vi "校准流程.vi"(0 "校准模式":T3(ring), 5 "参数下拉列表":u16(ring) items=["总氮"=1, "总磷"=2], 7 "测量模式":T1(ring), 9 "量程下拉列表":enum16{"低量程", "高量程"}(ring), 11 "曲线模型":T2={"标液浓度1"=0.0, "测量吸光度1"=0.0, "样品1启用"=FALSE, "标液浓度2"=0.0, "测量吸光度2"=0.0, "样品2启用"=FALSE, "标液浓度3"=0.0, "测量吸光度3"=0.0, "样品3启用"=FALSE, "标液浓度4"=0.0, "测量吸光度4"=0.0, "样品4启用"=FALSE, "标液浓度5"=0.0, "测量吸光度5"=0.0, "样品5启用"=FALSE, "模型"=enum."线性", "精度"=4.0, "XY图"=[], "拟合公式"="", "r^2"=0.0, "标样一校准时间"=timestamp(0 s since 1904-01-01), "标样二校准时间"=timestamp(0 s since 1904-01-01), "标样三校准时间"=timestamp(0 s since 1904-01-01), "标样四校准时间"=timestamp(0 s since 1904-01-01), "标样五校准时间"=timestamp(0 s since 1904-01-01), "二次方程"={"c"=0.0, "x"=0.0, "x^2"=0.0}, "标定时间"=timestamp(0 s since 1904-01-01)} {"标定时间" format="%<%m/%d/%y %H:%M:%S>T"; "标样五校准时间" format="%<%m/%d/%y %H:%M:%S>T"; "标样四校准时间" format="%<%m/%d/%y %H:%M:%S>T"; "标样三校准时间" format="%<%m/%d/%y %H:%M:%S>T"; "标样二校准时间" format="%<%m/%d/%y %H:%M:%S>T"; "标样一校准时间" format="%<%m/%d/%y %H:%M:%S>T"; "r^2" format="%.7f"; "测量吸光度5" format="%#.6f"; "测量吸光度4" format="%#.6f"; "测量吸光度3" format="%#.6f"; "测量吸光度2" format="%#.6f"; "测量吸光度1" format="%#.6f"}) -> ()   [LabVIEW 2016, in "斯坦道总磷.lvlib"]
panel:
  out "输出簇":cluster{"数据时间":timestamp, "X值":sgl}
  # "校准时间"
  # "标液浓度"
  # "吸光值显示"
  # "标液一"
  # "标液二"
  # "标液三"
  # "零点"
  # "跨度"
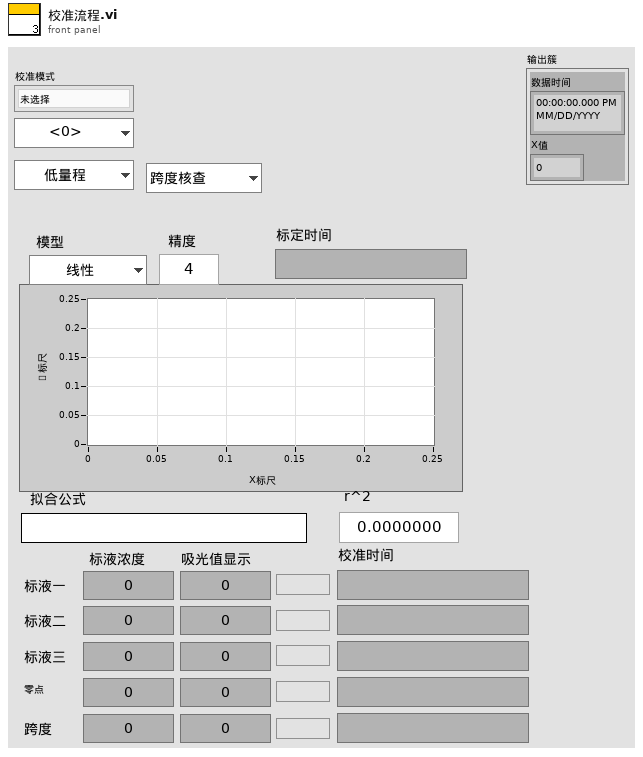
[diagram p1: front panel]
types:
  T1 = enum16{"跨度核查", "水样测量", "零点核查", "标样核查", "加标回收", "快捷测试", "空白校准", "标样校准"}
  T2 = cluster{"标液浓度1":dbl, "测量吸光度1":dbl, "样品1启用":bool, "标液浓度2":dbl, "测量吸光度2":dbl, "样品2启用":bool, "标液浓度3":dbl, "测量吸光度3":dbl, "样品3启用":bool, "标液浓度4":dbl, "测量吸光度4":dbl, "样品4启用":bool, "标液浓度5":dbl, "测量吸光度5":dbl, "样品5启用":bool, "模型":enum32{"线性", "多项式"}, "精度":dbl, "XY图":cluster{"X Values":dbl[], "Y Values":dbl[]}[], "拟合公式":string, "r^2":dbl, "标样一校准时间":timestamp, "标样二校准时间":timestamp, "标样三校准时间":timestamp, "标样四校准时间":timestamp, "标样五校准时间":timestamp, "二次方程":cluster{"c":dbl, "x":dbl, "x^2":dbl}, "标定时间":timestamp}
  T3 = enum32{"未选择", "空白校准", "标样校准", "标样核查", "零点核查", "跨度核查"}
  T4 = enum16{"初始化", "校准启动", "校准运行中", "测试结束", "获取校准数据", "填充校准数据", "流程结束"}
  T5 = enum16{"空闲", "初始化", "校准启动", "校准运行中", "测试结束", "获取校准数据", "填充校准数据", "流程结束"}
  T6 = cluster{"站号":u16, "量程切换":enum32{"H", "L", "AUTO"}, "控制命令":enum16{"启动测量", "标样核查", "零点核查", "跨度核查", "空白测试", "平行样测试", "加标回收", "空白校准", "标样校准", "初始化（清洗）", "停止测试", "仪器重启", "校时", "模式设置", "测量间隔设置"}, "模式设置":enum16{"待机", "连续模式", "周期模式", "定点模式", "受控模式", "手动模式"}, "测量间隔":u16}
  T7 = enum16{"启动测量", "标样核查", "零点核查", "跨度核查", "空白测试", "平行样测试", "加标回收", "空白校准", "标样校准", "初始化（清洗）", "停止测试", "仪器重启", "校时", "模式设置", "测量间隔设置"}
  T8 = cluster{"因子编码":u32, "单位":u16, "标样参考值":sgl, "水样数据时间":timestamp, "水样实测值":sgl, "水样数据标识":string, "标样数据时间":timestamp, "标样实测值":sgl, "标样数据标识":string, "空白数据时间":timestamp, "空白实测值":sgl, "空白数据标识":string, "零点核查数据时间":timestamp, "零点核查实测值":sgl, "零点核查数据标识":string, "跨度核查数据时间":timestamp, "跨度核查实测值":sgl, "跨度核查数据标识":string, "加标回收数据时间":timestamp, "加标回收实测值":sgl, "加标回收数据标识":string, "平行样数据时间":timestamp, "平行样实测值":sgl, "平行样数据标识":string, "F0":sgl, "F1":sgl, "F2":sgl, "F3":sgl, "F4":sgl, "F5":sgl, "F6":sgl, "F7":sgl, "温度":sgl, "湿度":sgl, "X值":sgl, "fidrange":u16, "X1值":sgl}
  T9 = cluster{"系统时间":timestamp, "工作状态":u16, "测量模式":enum16{"待机", "连续模式", "周期模式", "定点模式", "受控模式", "手动模式"}, "告警代码":u16, "故障代码":u16, "日志代码":u16, "软件版本":u16, "F0":sgl, "F1":sgl, "F2":sgl, "F3":sgl, "T":sgl, "H":sgl, "id":u16, "flowid":u16, "量程":u16, "总磷控温温度1":sgl, "营养盐控温温度2":sgl, "ADC":sgl, "结果值":sgl, "运行时间":u16, "步骤详情":string, "步骤流程":string}
  T10 = cluster{"标液浓度1":dbl, "测量吸光度1":dbl, "样品1启用":bool, "标液浓度2":dbl, "测量吸光度2":dbl, "样品2启用":bool, "标液浓度3":dbl, "测量吸光度3":dbl, "样品3启用":bool, "标液浓度4":dbl, "测量吸光度4":dbl, "样品4启用":bool, "标液浓度5":dbl, "测量吸光度5":dbl, "样品5启用":bool, "模型":enum32{"线性", "多项式"}, "精度":dbl, "XY图":cluster{"X Values":dbl[], "Y Values":dbl[]}[], "拟合公式":string, "r^2":dbl, "标样一校准时间":timestamp, "标样二校准时间":timestamp, "标样三校准时间":timestamp, "标样四校准时间":timestamp, "标样五校准时间":timestamp, "二次方程":cluster{"c":dbl, "x":dbl, "x^2":dbl}, "标定时间":timestamp}[]
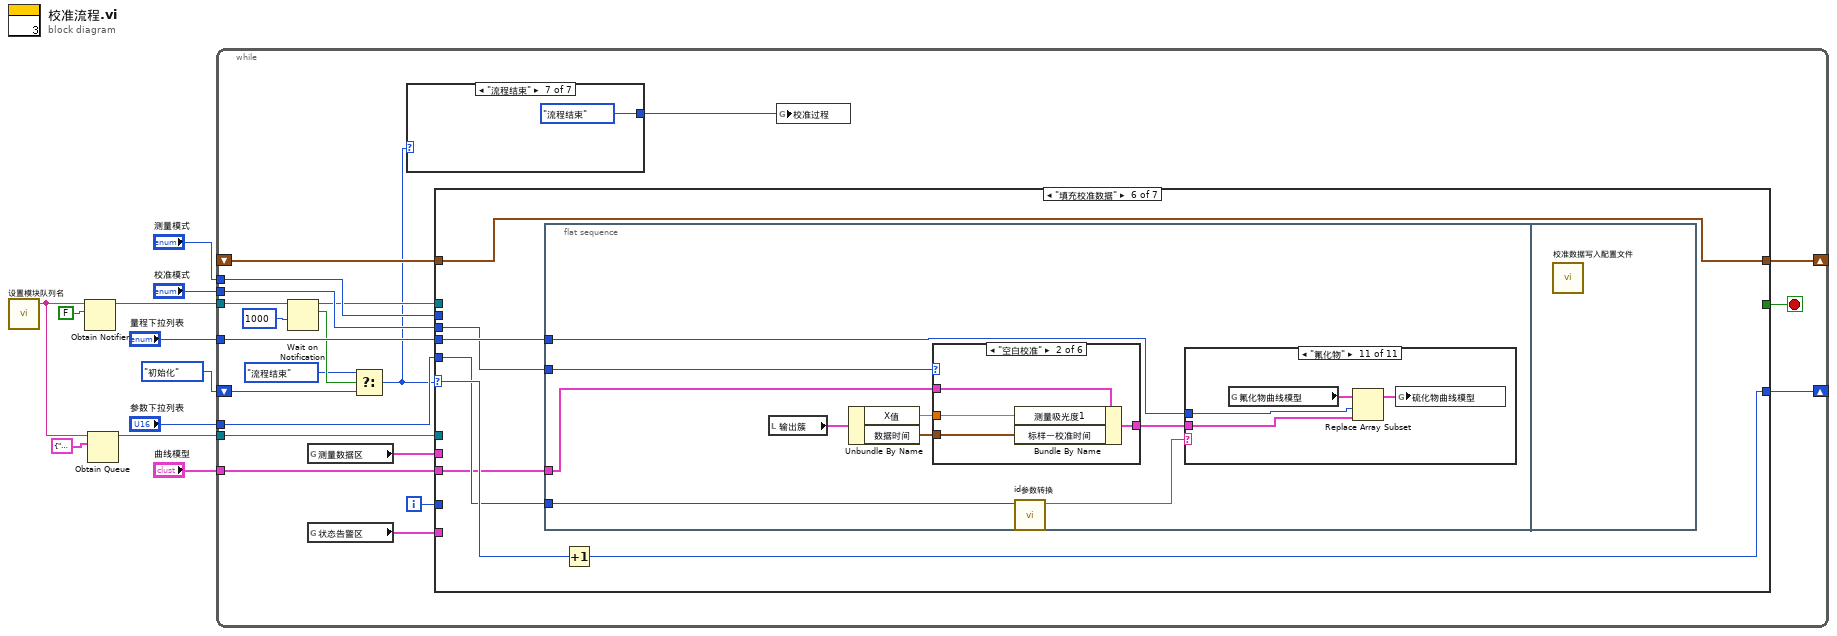
[diagram p0: block diagram]
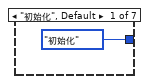
[diagram p2: hidden frame]
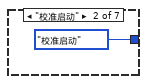
[diagram p3: hidden frame]
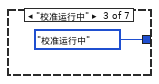
[diagram p4: hidden frame]
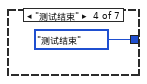
[diagram p5: hidden frame]
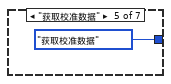
[diagram p6: hidden frame]
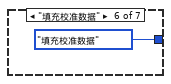
[diagram p7: hidden frame]
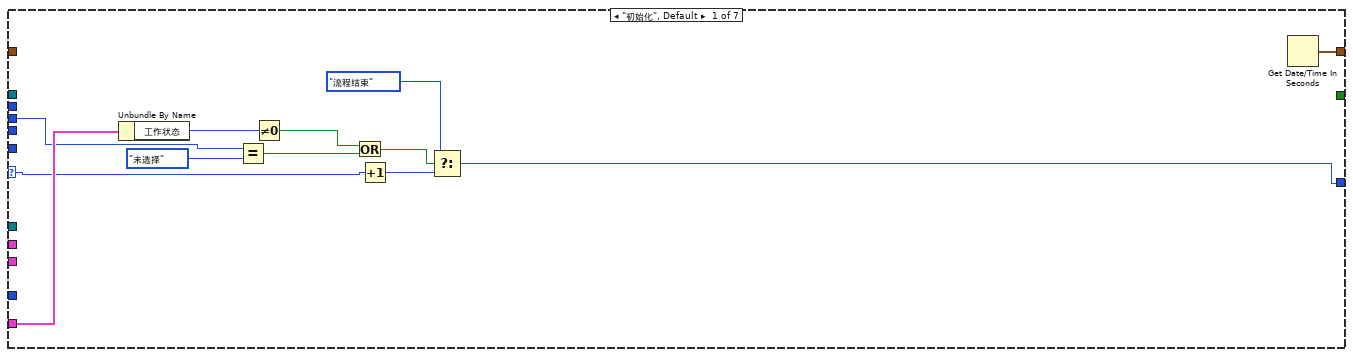
[diagram p8: hidden frame]
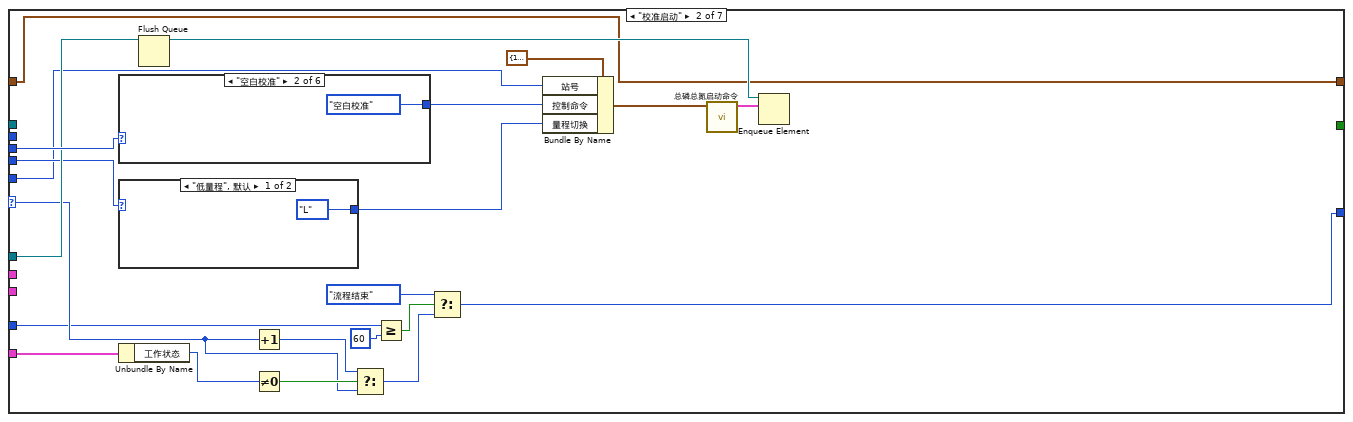
[diagram p9: hidden frame]
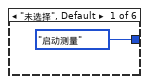
[diagram p10: hidden frame]
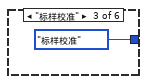
[diagram p11: hidden frame]
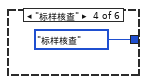
[diagram p12: hidden frame]
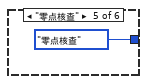
[diagram p13: hidden frame]
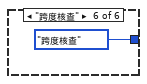
[diagram p14: hidden frame]
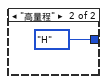
[diagram p15: hidden frame]
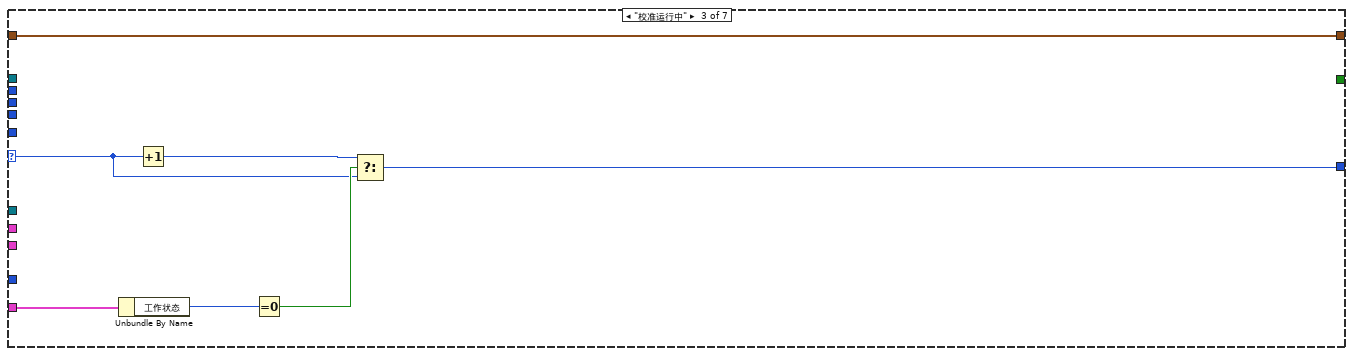
[diagram p16: hidden frame]
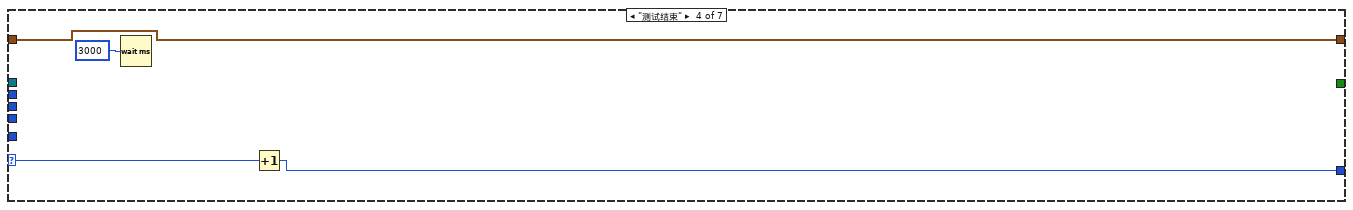
[diagram p17: hidden frame]
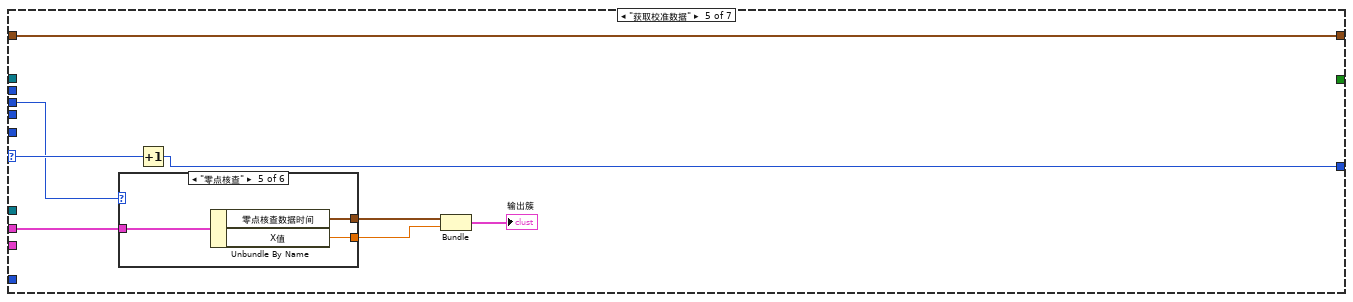
[diagram p18: hidden frame]
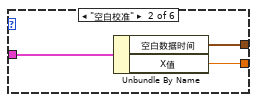
[diagram p20: hidden frame]
diagram:
  n1 = call "设置模块队列名.vi"() -> ("Msg"=w2:string)  [unwired: 5 in]
  n2 = Obtain Notifier(name (unnamed)=w2, notification data type=FALSE) -> (notifier out=w1:refnum<notifier>)  [unwired: 2 in, 2 out]
  n3 = Obtain Queue(name (unnamed)=w2, element data type=cluster{"命令":string, "data":variant} {"命令"="", "data"=variant}) -> (queue out=w8:refnum<queue>)  [unwired: 3 in, 2 out]
  n4 = while {
    tunnel: "校准模式" -> [w31]
    shift-right: [w29] -> _
    shift-left: T4."初始化" ("枚举") -> [w16]
    tunnel: w8 -> [w32]
    tunnel: "量程下拉列表" -> [w28]
    tunnel: "参数下拉列表" -> [w27]
    shift-right: [w26] -> _
    shift-left: _ -> [w25]
    tunnel: "曲线模型" -> [w22]
    tunnel: "测量模式" -> [w21]
    tunnel: w1 -> [w19]
    i -> [w20]
    stop <- w30 stop-if-true
    n5 = Wait on Notification(notifier=w19, timeout in ms (-1)=1000 ("超时毫秒(-1)")) -> (notifier out=w14:refnum<notifier>, notification=w17:bool)  [unwired: 2 in, 2 out]
    n6 = global read "VAR总磷总氮全局变量.vi" "测量数据区"() -> (w24:T8)
    n7 = global read "VAR总磷总氮全局变量.vi" "状态告警区"() -> (w23:T9)
    n8 = Select(t=T4."流程结束", s=w17, f=w16) -> (s? t:f=w13:T4)
    n9 = case shown="\"流程结束\"" w13 {
      tunnel: [T5."初始化" ("校准过程") T5."校准启动" ("校准过程") T5."校准运行中" ("校准过程") T5."测试结束" ("校准过程") T5."获取校准数据" ("校准过程") T5."填充校准数据" ("校准过程") T5."流程结束" ("校准过程")] -> w12
      frame "初始化", Default {
      }
      frame "校准启动" {
      }
      frame "校准运行中" {
      }
      frame "测试结束" {
      }
      frame "获取校准数据" {
      }
      frame "填充校准数据" {
      }
      frame "流程结束" {
      }
    }
    n10 = case shown="\"填充校准数据\"" w13 {
      selector: w13 -> [w47 w59 w87 w92 w100 w122 w195]
      tunnel: w32 -> [_ w66 _ _ _ _ w193]
      tunnel: w31 -> [w43 w67 _ _ w98 w117 _]
      tunnel: [_ _ _ _ _ _ TRUE] -> w30
      tunnel: [w45 w53 w85 w90 w95 w116 w195] -> w29
      tunnel: w28 -> [_ w65 _ _ _ w119 _]
      tunnel: w27 -> [_ w64 _ _ _ w120 _]
      tunnel: w23 -> [w50 w62 w83 _ _ _ _]
      tunnel: [w51 w63 w84 w91 w93 w121 w194] -> w26
      tunnel: w25 -> [_ w63 w84 w91 w93 w121 w194]
      tunnel: w24 -> [_ _ _ _ w99 _ _]
      tunnel: w22 -> [_ _ _ _ _ w118 _]
      tunnel: w21 -> [_ _ _ _ _ _ _]
      tunnel: w20 -> [_ w57 _ _ _ _ _]
      tunnel: w14 -> [_ _ _ _ _ _ w192]
      frame "初始化", Default {
        n11 = Unbundle By Name(w50) -> ("工作状态"=w49:u16)
        n12 = Equal?(x=w43, y=T3."未选择") -> (x = y?=w40:bool)
        n13 = Not Equal To 0?(x=w49) -> (x != 0?=w48:bool)
        n14 = Or(x=w48, y=w40) -> (x .or. y?=w41:bool)
        n15 = Increment(x=w47) -> (x+1=w46:T4)
        n16 = Select(t=T4."流程结束", s=w41, f=w46) -> (s? t:f=w45:T4)
        n17 = Get Date/Time In Seconds() -> (seconds since 1Jan1904=w51:timestamp)
      }
      frame "校准启动" {
        n18 = case shown="\"空白校准\"" w67 {
          tunnel: [T7."启动测量" ("控制命令") T7."空白校准" ("控制命令") T7."标样校准" ("控制命令") T7."标样核查" ("控制命令") T7."零点核查" ("控制命令") T7."跨度核查" ("控制命令")] -> w73
          frame "未选择", Default {
          }
          frame "空白校准" {
          }
          frame "标样校准" {
          }
          frame "标样核查" {
          }
          frame "零点核查" {
          }
          frame "跨度核查" {
          }
        }
        n19 = case shown="\"低量程\", 默认" w65 {
          tunnel: [enum32{"H", "L", "AUTO"}."L" ("量程切换") enum32{"H", "L", "AUTO"}."H" ("量程切换")] -> w72
          frame "低量程", Default {
          }
          frame "高量程" {
          }
        }
        n20 = Unbundle By Name(w62) -> ("工作状态"=w61:u16)
        n21 = Flush Queue(queue=w66) -> (queue out=w69:refnum<queue>)  [unwired: 1 in, 2 out]
        n22 = Increment(x=w59) -> (x+1=w58:T4)
        n23 = Not Equal To 0?(x=w61) -> (x != 0?=w60:bool)
        n24 = Select(t=w58, s=w60, f=w59) -> (s? t:f=w54:T4)
        n25 = Greater Or Equal?(x=w57, y=60) -> (x >= y?=w55:bool)
        n26 = Select(t=T4."流程结束", s=w55, f=w54) -> (s? t:f=w53:T4)
        n27 = Bundle By Name(cluster=T6 {"站号"=1, "量程切换"=enum."AUTO", "控制命令"=enum."启动测量", "模式设置"=enum."待机", "测量间隔"=0} ("参数"), "站号"=w64, "控制命令"=w73, "量程切换"=w72) -> (w71:T6)
        n28 = call "总磷总氮启动命令.vi"("参数"=w71) -> ("启动命令"=w68:cluster{"命令":string, "data":variant})  [unwired: 10 in]
        n29 = Enqueue Element(queue=w69, element=w68) -> ()  [unwired: 2 in, 3 out]
      }
      frame "校准运行中" {
        n30 = Unbundle By Name(w83) -> ("工作状态"=w82:u16)
        n31 = Increment(x=w87) -> (x+1=w86:T4)
        n32 = Equal To 0?(x=w82) -> (x = 0?=w88:bool)
        n33 = Select(t=w86, s=w88, f=w87) -> (s? t:f=w85:T4)
      }
      frame "测试结束" {
        n34 = Wait (ms)(milliseconds to wait=u32 3000 ("等待时间（毫秒）")) -> ()  [unwired: 1 out]
        n35 = Increment(x=w92) -> (x+1=w90:T4)
      }
      frame "获取校准数据" {
        n36 = case shown="\"零点核查\"" w98 {
          tunnel: w99 -> [_ w103 w106 w109 w112 w115]
          tunnel: [_ w102 w105 w108 w111 w114] -> w94
          tunnel: [_ w101 w104 w107 w110 w113] -> w97
          frame "未选择", Default {
          }
          frame "空白校准" {
            n37 = Unbundle By Name(w103) -> ("空白数据时间"=w102:timestamp, "X值"=w101:sgl)
          }
          frame "标样校准" {
            n38 = Unbundle By Name(w106) -> ("标样数据时间"=w105:timestamp, "X值"=w104:sgl)
          }
          frame "标样核查" {
            n39 = Unbundle By Name(w109) -> ("标样数据时间"=w108:timestamp, "X值"=w107:sgl)
          }
          frame "零点核查" {
            n40 = Unbundle By Name(w112) -> ("零点核查数据时间"=w111:timestamp, "X值"=w110:sgl)
          }
          frame "跨度核查" {
            n41 = Unbundle By Name(w115) -> ("跨度核查数据时间"=w114:timestamp, "X值"=w113:sgl)
          }
        }
        n42 = Increment(x=w100) -> (x+1=w95:T4)
        n43 = Bundle("跨度核查数据时间"=w94, "X值"=w97) -> (→"输出簇":cluster{"跨度核查数据时间":timestamp, "X值":sgl})  [unwired: 1 in]
      }
      frame "填充校准数据" {
        n44 = flat-sequence {
          tunnel: w120 -> [w130]
          tunnel: w119 -> [w129]
          tunnel: w118 -> [w128]
          tunnel: w117 -> [w126]
          frame #0 {
            n45 = local read "输出簇"() -> (w125:cluster{"数据时间":timestamp, "X值":sgl})
            n46 = Unbundle By Name(w125) -> ("X值"=w124:sgl, "数据时间"=w123:timestamp)
            n47 = case shown="\"空白校准\"" w126 {
              tunnel: w128 -> [_ w135 w139 w143 w147 w151]
              tunnel: [_ w134 w138 w142 w146 w150] -> w127
              tunnel: w124 -> [_ w133 w137 w141 w145 w149]
              tunnel: w123 -> [_ w132 w136 w140 w144 w148]
              frame "未选择", Default {
              }
              frame "空白校准" {
                n48 = Bundle By Name(cluster=w135, "测量吸光度1"=w133, "标样一校准时间"=w132) -> (w134:T2)
              }
              frame "标样校准" {
                n49 = Bundle By Name(cluster=w139, "测量吸光度2"=w137, "标样二校准时间"=w136) -> (w138:T2)
              }
              frame "标样核查" {
                n50 = Bundle By Name(cluster=w143, "测量吸光度3"=w141, "标样三校准时间"=w140) -> (w142:T2)
              }
              frame "零点核查" {
                n51 = Bundle By Name(cluster=w147, "测量吸光度4"=w145, "标样四校准时间"=w144) -> (w146:T2)
              }
              frame "跨度核查" {
                n52 = Bundle By Name(cluster=w151, "测量吸光度5"=w149, "标样五校准时间"=w148) -> (w150:T2)
              }
            }
            n53 = call "id参数转换.vi"("id"=w130) -> ("table输出"=w131:string)  [unwired: 9 in, 1 out]
            n54 = case shown="\"氟化物\"" w131 {
              tunnel: w127 -> [_ w155 w159 w162 w165 w169 w173 w177 w181 w186 w190]
              tunnel: w129 -> [_ w152 w156 w160 w164 w168 w172 w176 w180 w184 w188]
              frame Default {
              }
              frame "总磷" {
                n55 = global read "校准数据全局变量.vi" "总磷曲线模型"() -> (w153:T10)
                n56 = Replace Array Subset(array=w153, new element=w155, index=w152) -> (w154:T10)
                n57 = global write "校准数据全局变量.vi" "总磷曲线模型"(w154) -> ()
              }
              frame "总氮" {
                n58 = global read "校准数据全局变量.vi" "总氮曲线模型"() -> (w158:T10)
                n59 = Replace Array Subset(array=w158, new element=w159, index=w156) -> (w157:T10)
                n60 = global write "校准数据全局变量.vi" "总氮曲线模型"(w157) -> ()
              }
              frame "氨氮" {
                n61 = global read "校准数据全局变量.vi" "氨氮曲线模型"() -> (w163:T10)
                n62 = Replace Array Subset(array=w163, new element=w162, index=w160) -> (w161:T10)
                n63 = global write "校准数据全局变量.vi" "氨氮曲线模型"(w161) -> ()
              }
              frame "磷酸盐" {
                n64 = global read "校准数据全局变量.vi" "磷酸盐曲线模型"() -> (w167:T10)
                n65 = Replace Array Subset(array=w167, new element=w165, index=w164) -> (w166:T10)
                n66 = global write "校准数据全局变量.vi" "磷酸盐曲线模型"(w166) -> ()
              }
              frame "硝氮" {
                n67 = global read "校准数据全局变量.vi" "硝氮曲线模型"() -> (w171:T10)
                n68 = Replace Array Subset(array=w171, new element=w169, index=w168) -> (w170:T10)
                n69 = global write "校准数据全局变量.vi" "硝氮曲线模型"(w170) -> ()
              }
              frame "亚硝氮" {
                n70 = global read "校准数据全局变量.vi" "亚硝氮曲线模型"() -> (w175:T10)
                n71 = Replace Array Subset(array=w175, new element=w173, index=w172) -> (w174:T10)
                n72 = global write "校准数据全局变量.vi" "亚硝氮曲线模型"(w174) -> ()
              }
              frame "硅酸盐" {
                n73 = global read "校准数据全局变量.vi" "硅酸盐曲线模型"() -> (w179:T10)
                n74 = Replace Array Subset(array=w179, new element=w177, index=w176) -> (w178:T10)
                n75 = global write "校准数据全局变量.vi" "硅酸盐曲线模型"(w178) -> ()
              }
              frame "硫化物" {
                n76 = global read "校准数据全局变量.vi" "硫化物曲线模型"() -> (w183:T10)
                n77 = Replace Array Subset(array=w183, new element=w181, index=w180) -> (w182:T10)
                n78 = global write "校准数据全局变量.vi" "硫化物曲线模型"(w182) -> ()
              }
              frame "CODcr" {
                n79 = global read "校准数据全局变量.vi" "CODcr曲线模型"() -> (w187:T10)
                n80 = Replace Array Subset(array=w187, new element=w186, index=w184) -> (w185:T10)
                n81 = global write "校准数据全局变量.vi" "CODcr曲线模型"(w185) -> ()
              }
              frame "氟化物" {
                n82 = global read "校准数据全局变量.vi" "氟化物曲线模型"() -> (w191:T10)
                n83 = Replace Array Subset(array=w191, new element=w190, index=w188) -> (w189:T10)
                n84 = global write "校准数据全局变量.vi" "硫化物曲线模型"(w189) -> ()
              }
            }
          }
          frame #1 {
            n85 = call "校准数据写入配置文件.vi"() -> ()  [unwired: 11 in, 1 out]
          }
        }
        n86 = Increment(x=w122) -> (x+1=w116:T4)
      }
      frame "流程结束" {
        n87 = Release Notifier(notifier=w192) -> ()  [unwired: 2 in, 3 out]
        n88 = Release Queue(queue=w193) -> ()  [unwired: 2 in, 3 out]
      }
    }
    n89 = global write "VAR总磷总氮全局变量.vi" "校准过程"(w12) -> ()
  }
